vi "Stitching-Calculate image location in pixels.vi"(9 "FOV (um)":dbl=175.0, 10 "Image location (um)":dbl=350.0, 11 "Single image size (pixels)":i32=512) -> (3 "image location within canvas (pixels)":i32)   [LabVIEW 2020]
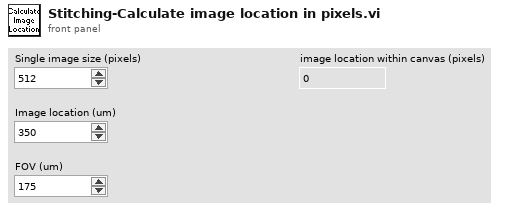
[diagram p1: front panel]
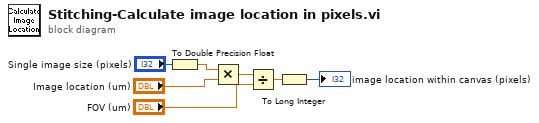
[diagram p0: block diagram]
diagram:
  n1 = To Double Precision Float(number="Single image size (pixels)") -> (double precision float=w2:dbl)
  n2 = Multiply(x=w2, y="Image location (um)") -> (x*y=w5:dbl)
  n3 = Divide(x=w5, y="FOV (um)") -> (x/y=w7:dbl)
  n4 = To Long Integer(number=w7) -> (32bit integer=→"image location within canvas (pixels)":i32)
